vi "Highlight Rows By Category.vi"(8 "error in (no error)":errorcluster, 10 "Category Name":string, 11 "MulticolumnListbox in":refnum<vi>) -> (0 "error out":errorcluster)   [LabVIEW 2018]
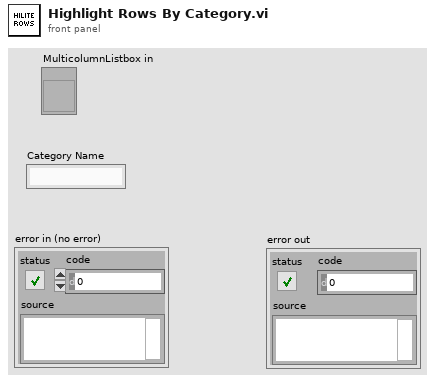
[diagram p1: front panel]
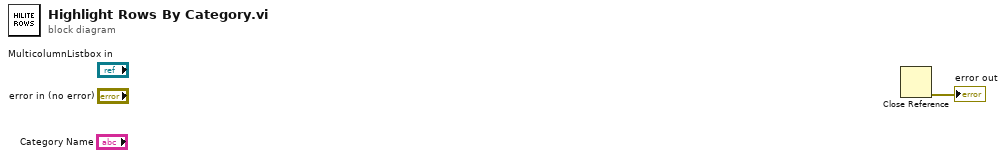
[diagram p0: block diagram]
diagram:
  n1 = Close Reference() -> (error out=→"error out":errorcluster)  [unwired: 2 in]
